vi "Untitled 1 (SubVI).vi"(8 "D gain":dbl, 9 "I gain":dbl, 10 "P gain":dbl, 11 "Numeric in":dbl) -> (3 "Numeric out":dbl)   [LabVIEW 2019]
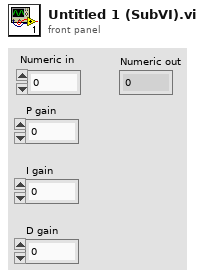
[diagram p1: front panel]
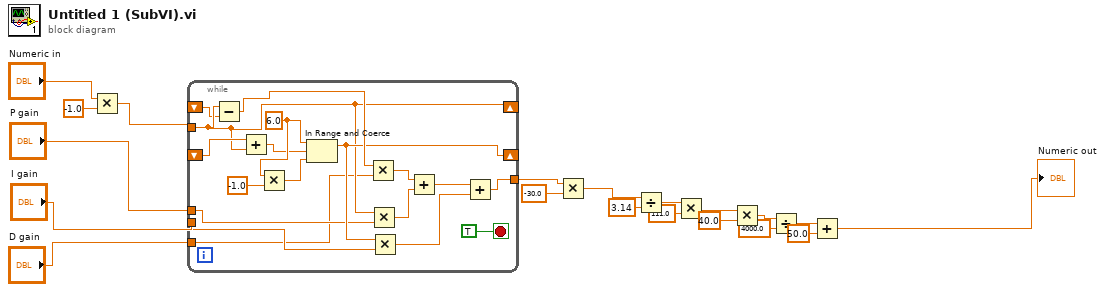
[diagram p0: block diagram]
diagram:
  n1 = Multiply(x="Numeric in", y=-1.0) -> (x*y=w18:dbl)
  n2 = while {
    shift-right: [w30] -> _
    shift-left: _ -> [w36]
    tunnel: w18 -> [w24]
    shift-right: [w24] -> _
    shift-left: _ -> [w23]
    tunnel: "P gain" -> [w22]
    tunnel: "I gain" -> [w21]
    tunnel: "D gain" -> [w20]
    tunnel: [w25] -> w12
    stop <- TRUE stop-if-true
    w33 = 6.0 ("upper limit")
    n3 = Subtract(x=w24, y=w23) -> (x-y=w31:dbl)
    n4 = Add(x=w36, y=w24) -> (x+y=w32:dbl)
    n5 = Multiply(x=w33, y=-1.0) -> (x*y=w34:dbl)
    n6 = In Range and Coerce(upper limit=w33, x=w32, lower limit=w34) -> (coerced(x)=w30:dbl)  [unwired: 1 out]
    n7 = Multiply(x=w31, y=w20) -> (x*y=w29:dbl)
    n8 = Multiply(x=w24, y=w22) -> (x*y=w28:dbl)
    n9 = Multiply(x=w30, y=w21) -> (x*y=w26:dbl)
    n10 = Add(x=w29, y=w28) -> (x+y=w27:dbl)
    n11 = Add(x=w27, y=w26) -> (x+y=w25:dbl)
  }
  n12 = Multiply(x=w12, y=-30.0) -> (x*y=w11:dbl)
  n13 = Divide(x=w11, y=3.14) -> (x/y=w9:dbl)
  n14 = Multiply(x=w9, y=111.0) -> (x*y=w7:dbl)
  n15 = Multiply(x=w7, y=40.0) -> (x*y=w5:dbl)
  n16 = Divide(x=w5, y=4000.0) -> (x/y=w3:dbl)
  n17 = Add(x=w3, y=50.0) -> (x+y=→"Numeric out":dbl)
